vi "BLOCK (SubVI).vi"(9 "reference 3":refnum<vi>, 10 "reference in":refnum<vi>, 11 "Digital in":refnum<vi>) -> (3 "Array":bool[](array[boolean]))   [LabVIEW 2021]
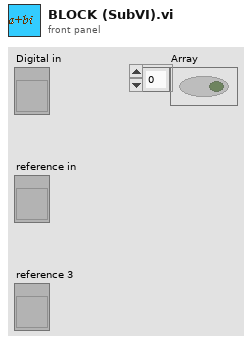
[diagram p1: front panel]
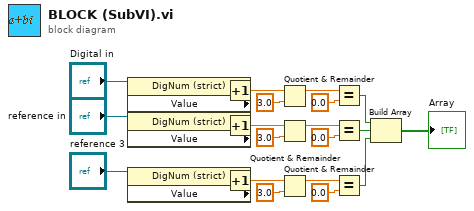
[diagram p0: block diagram]
diagram:
  n1 = property class="DigNum (strict)"(reference="Digital in") -> ("Value"=w20:dbl)  [unwired: 1 in, 2 out]
  n2 = property class="DigNum (strict)"(reference="reference in") -> ("Value"=w21:dbl)  [unwired: 1 in, 2 out]
  n3 = property class="DigNum (strict)"(reference="reference 3") -> ("Value"=w22:dbl)  [unwired: 1 in, 2 out]
  n4 = Increment(x=w20) -> (x+1=w17:dbl)
  n5 = Increment(x=w21) -> (x+1=w18:dbl)
  n6 = Increment(x=w22) -> (x+1=w19:dbl)
  n7 = Quotient & Remainder(x=w17, y=3.0) -> (x-y*floor(x/y)=w16:dbl)  [unwired: 1 out]
  n8 = Quotient & Remainder(x=w18, y=3.0) -> (x-y*floor(x/y)=w15:dbl)  [unwired: 1 out]
  n9 = Quotient & Remainder(x=w19, y=3.0) -> (x-y*floor(x/y)=w14:dbl)  [unwired: 1 out]
  n10 = Equal?(x=w16, y=0.0) -> (x = y?=w6:bool)
  n11 = Equal?(x=w15, y=0.0) -> (x = y?=w7:bool)
  n12 = Equal?(x=w14, y=0.0) -> (x = y?=w10:bool)
  n13 = Build Array(w6, w7, w10) -> (→"Array":bool[])
